vi "Add Item.vi"(3 "Error in":errorcluster, 5 "Item":u32) -> (0 "Error out":errorcluster)   [LabVIEW 2020]
uses:
  <vilib>/Utility/config.llb/NI_LVConfig.lvlib
  <vilib>/Utility/config.llb/Write Key (String).vi
panel:
  in  "Description":string
  in  "Access Level":enum16{"read-only", "write-only", "read/write"}(ring)
  in  "Data Type":enum16{"Double"}(ring)
  in  "Name":string
  in  "Cancel Button":bool
  in  "OK Button":bool
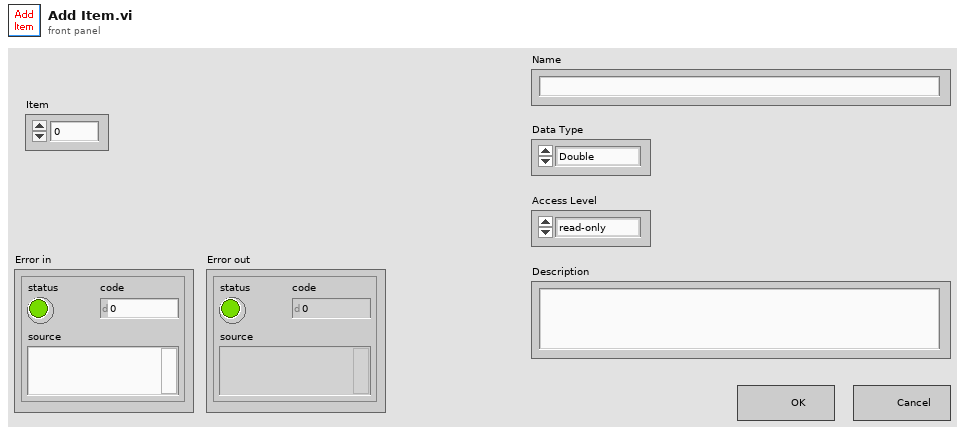
[diagram p1: front panel]
types:
  T1 = typedef "NI_LVConfig.lvlib/Config Data RefNum.ctl" = refnum<k1>
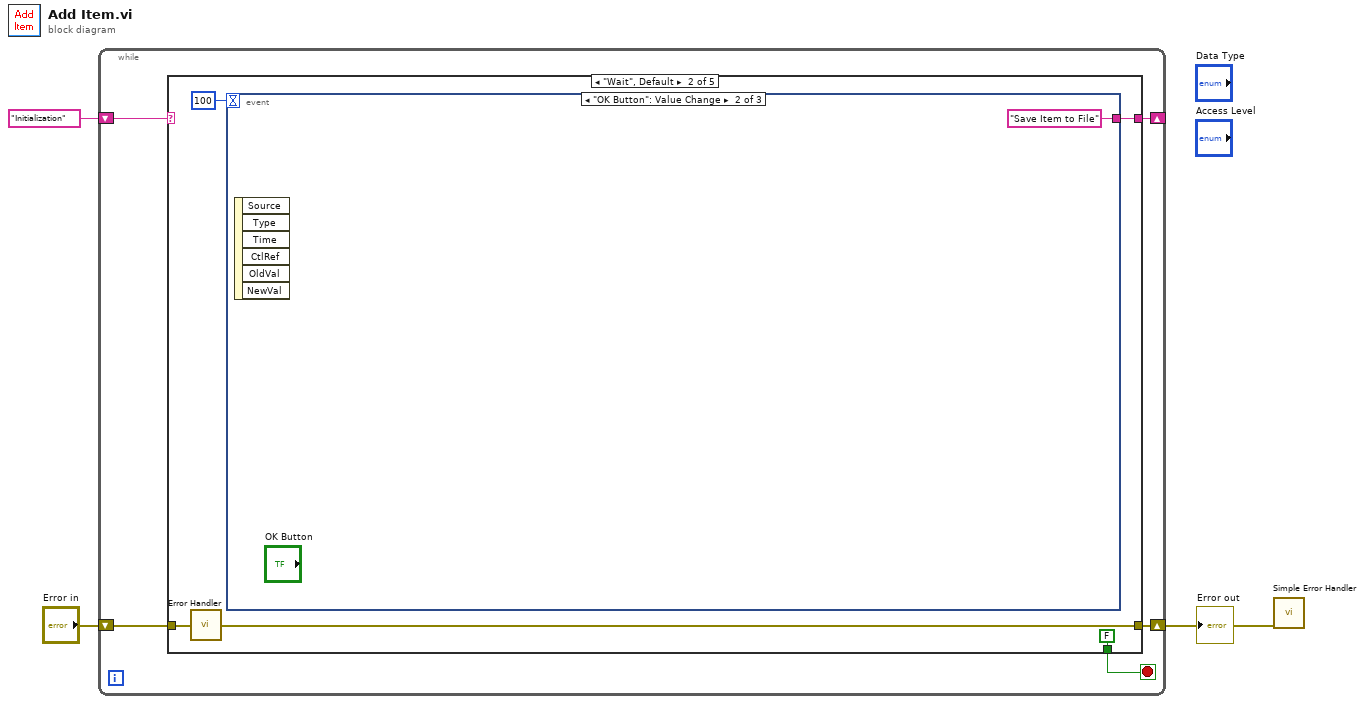
[diagram p0: block diagram]
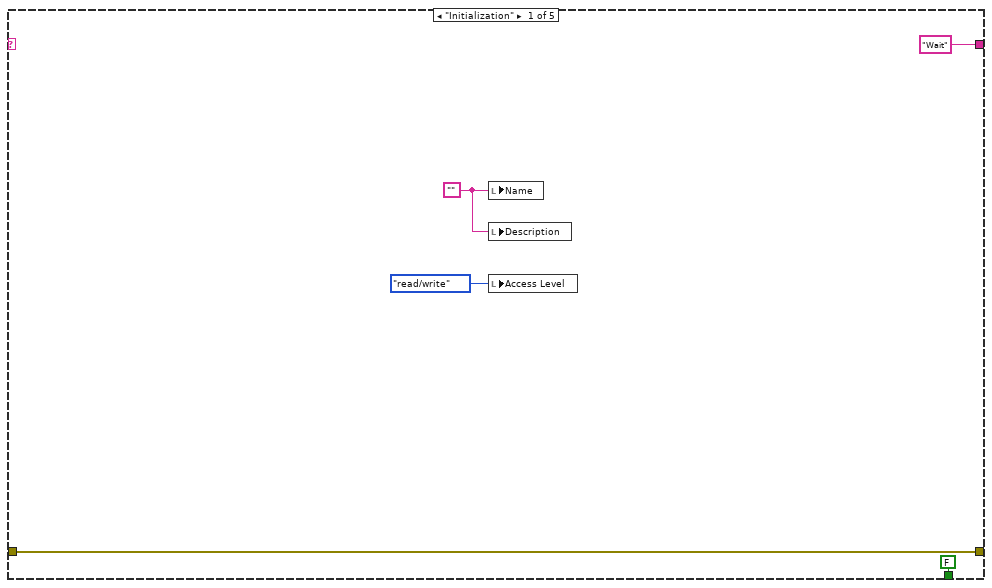
[diagram p2: hidden frame]
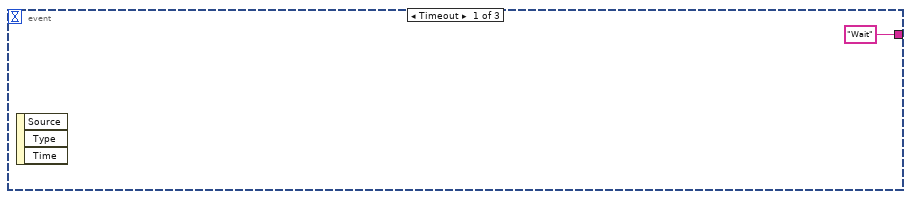
[diagram p3: hidden frame]
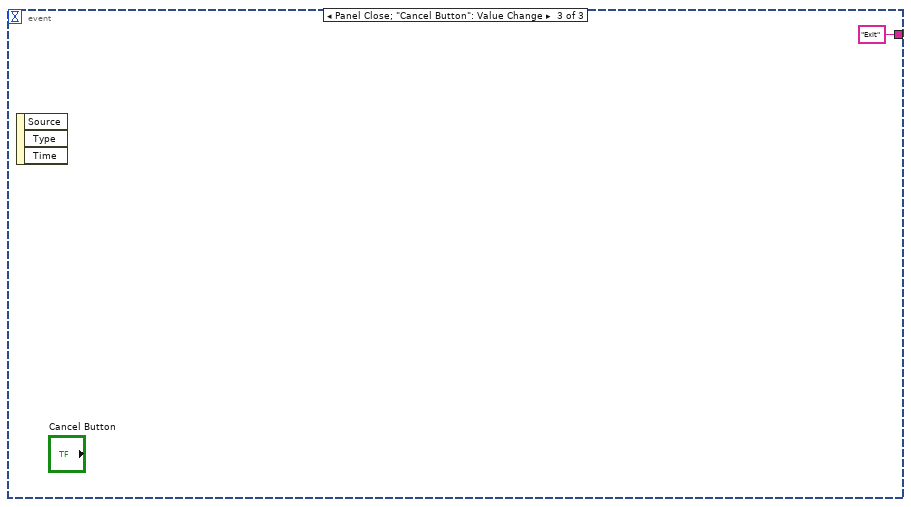
[diagram p4: hidden frame]
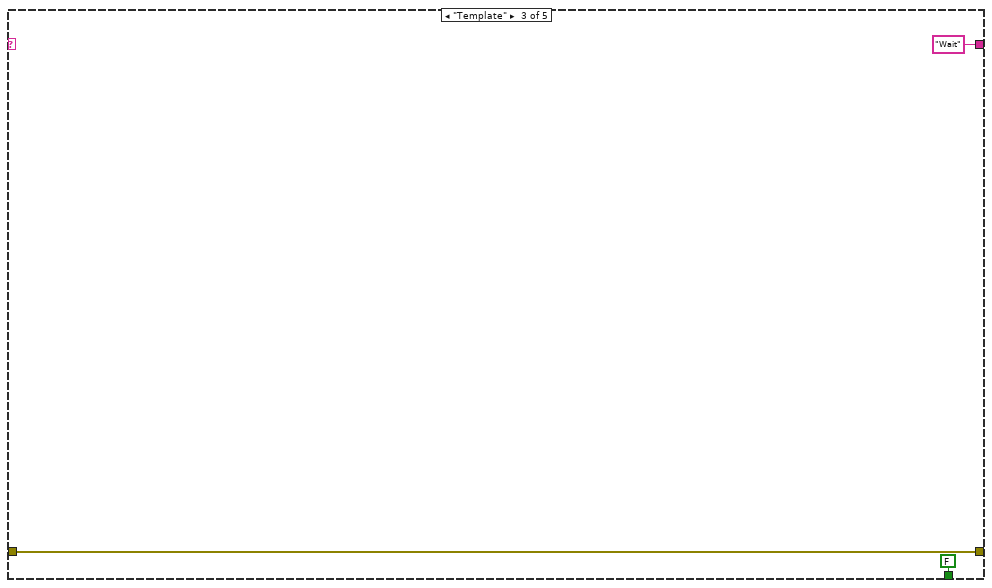
[diagram p5: hidden frame]
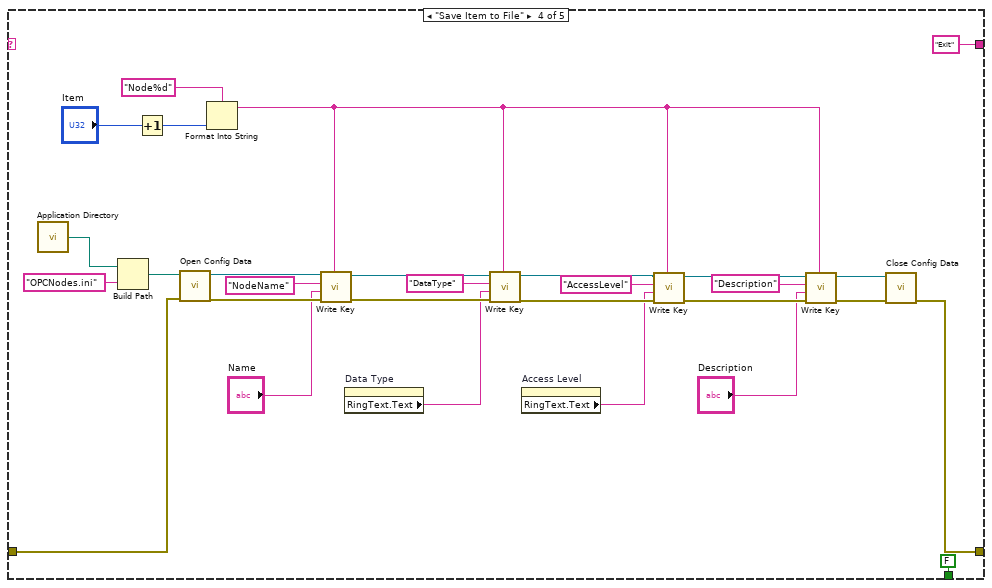
[diagram p6: hidden frame]
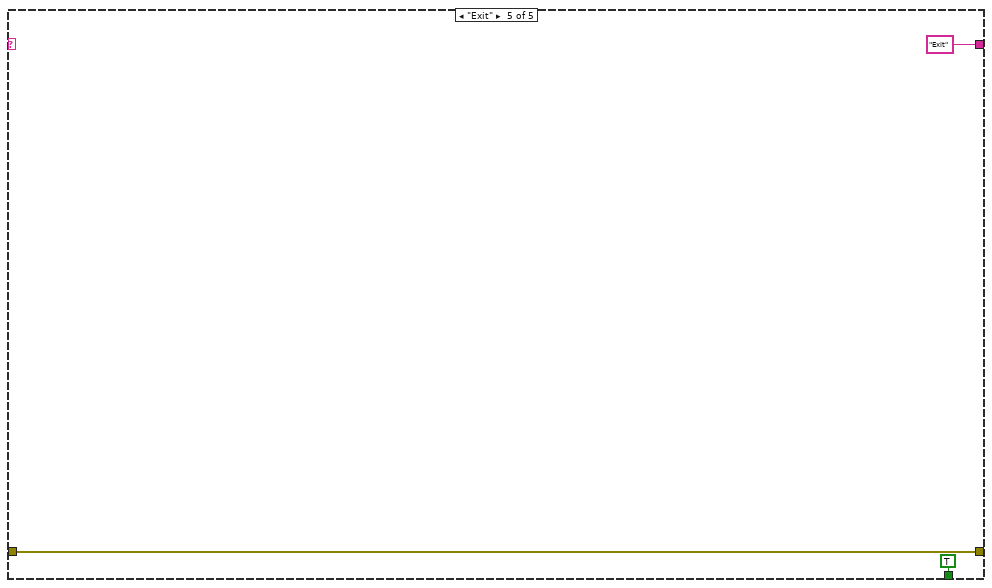
[diagram p7: hidden frame]
diagram:
  n1 = while {
    shift-right: [w7] -> _
    shift-left: "Initialization" -> [w8]
    shift-right: [w4] -> w1
    shift-left: "Error in" -> [w5]
    stop <- w6 stop-if-true
    n2 = case shown="\"Wait\", Default" w8 {
      tunnel: ["Wait" w16 "Wait" "Exit" "Exit"] -> w7
      tunnel: [FALSE FALSE FALSE FALSE TRUE] -> w6
      tunnel: w5 -> [w11 w14 w22 w33 w54]
      tunnel: [w11 w15 w22 w29 w54] -> w4
      frame "Initialization" {
        w9 = ""
        n3 = local write "Name"(w9) -> ()
        n4 = local write "Description"(w9) -> ()
        n5 = local write "Access Level"(enum16{"read-only", "write-only", "read/write"}."read/write" ("Access Level")) -> ()
      }
      frame "Wait", Default {
        n6 = call "Error Handler.vi"("Error in"=w14) -> ("Error out"=w15:errorcluster)
        n7 = event shown="[1] \"OK Button\": Value Change" {
          selector: _ -> [_ _ _]
          dyn-events: _ -> [_ _ _]
          timeout: 100 ("ms") -> [_ _ _]
          tunnel: ["Wait" "Save Item to File" "Exit"] -> w16
          event Timeout {
            n8 = event-data() -> ()  [unwired: 1 in, 3 out]
          }
          event "OK Button": Value Change {
            n9 = event-data() -> ()  [unwired: 1 in, 6 out]
          }
          event Panel Close; "Cancel Button": Value Change {
            n10 = event-data() -> ()  [unwired: 1 in, 3 out]
          }
        }
      }
      frame "Template" {
      }
      frame "Save Item to File" {
        n11 = call <vilib>:"Application Directory.vi"() -> ("Application Directory"=w51:path)
        n12 = Build Path(base path=w51, name or relative path="OPCNodes.ini") -> (appended path=w49:path)
        n13 = Increment(x="Item") -> (x+1=w26:u32)
        n14 = call <vilib>:"Open Config Data.vi"("error in (no error)"=w33, "configuration file path"=w49) -> ("error out"=w43:errorcluster, "refnum"=w48:T1)  [unwired: 7 in, 1 out]
        n15 = Format Into String(format string="Node%d" ("section"), w26) -> (resulting string=w25:string)  [unwired: 2 in, 1 out]
        n16 = call-poly <vilib>:"Write Key.vi"("section"=w25, "error in (no error)"=w43, "value"="Name", "key"="NodeName", "refnum"=w48) -> ("error out"=w42:errorcluster, "refnum out"=w36:T1)  [unwired: 4 in, 1 out]
        n17 = property on="Data Type" class="Enum (strict)"() -> ("RingText.Text"=w38:string)  [unwired: 2 in, 2 out]
        n18 = call-poly <vilib>:"Write Key.vi"("section"=w25, "error in (no error)"=w42, "value"=w38, "key"="DataType", "refnum"=w36) -> ("error out"=w41:errorcluster, "refnum out"=w35:T1)  [unwired: 4 in, 1 out]
        n19 = property on="Access Level" class="Enum (strict)"() -> ("RingText.Text"=w37:string)  [unwired: 2 in, 2 out]
        n20 = call-poly <vilib>:"Write Key.vi"("section"=w25, "error in (no error)"=w41, "value"=w37, "key"="AccessLevel", "refnum"=w35) -> ("error out"=w40:errorcluster, "refnum out"=w34:T1)  [unwired: 4 in, 1 out]
        n21 = call-poly <vilib>:"Write Key.vi"("section"=w25, "error in (no error)"=w40, "value"="Description", "key"="Description", "refnum"=w34) -> ("error out"=w30:errorcluster, "refnum out"=w31:T1)  [unwired: 4 in, 1 out]
        n22 = call <vilib>:"Close Config Data.vi"("error in (no error)"=w30, "refnum"=w31) -> ("error out"=w29:errorcluster)  [unwired: 8 in, 1 out]
      }
      frame "Exit" {
      }
    }
  }
  "Error out" <- w1
  n23 = call <vilib>:"Simple Error Handler.vi"("error in (no error)"=w1) -> ()  [unwired: 4 in, 5 out]
